vi "Find_Intersection.vi"(9 "line 2":cluster{"slope":dbl, "b":dbl, "theta":dbl}, 10 "line 1":cluster{"slope":dbl, "b":dbl, "theta":dbl}) -> (2 "Intersection":cluster{"x":dbl, "y":dbl})   [LabVIEW 2022 SP3]
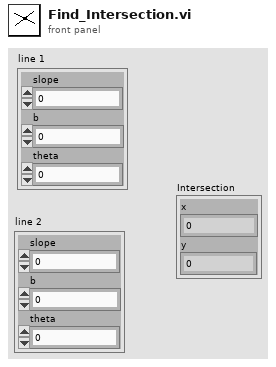
[diagram p1: front panel]
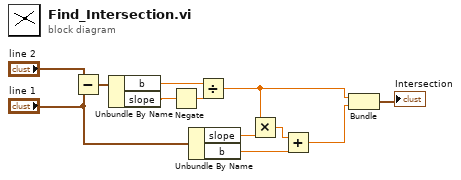
[diagram p0: block diagram]
diagram:
  n1 = Subtract(x="line 2", y="line 1") -> (x-y=w11:cluster{"slope":dbl, "b":dbl, "theta":dbl})
  n2 = Unbundle By Name(w11) -> ("b"=w10:dbl, "slope"=w9:dbl)
  n3 = Negate(x=w9) -> (-x=w8:dbl)
  n4 = Unbundle By Name("line 1") -> ("slope"=w6:dbl, "b"=w4:dbl)
  n5 = Divide(x=w10, y=w8) -> (x/y=w3:dbl)
  n6 = Multiply(x=w3, y=w6) -> (x*y=w5:dbl)
  n7 = Add(x=w5, y=w4) -> (x+y=w2:dbl)
  n8 = Bundle(w3, w2) -> (→"Intersection":cluster{dbl, dbl})  [unwired: 1 in]
